vi "Measurement Logic.vi"() -> ()   [LabVIEW 2021, in "Efficiency_Class D Amplifier.lvlib"]
uses:
  Efficiency_Class D Amplifier.lvlib
  Measurement Configuration.ctl
  shared/controls/digital audio protocol/data justification.ctl
  shared/controls/digital audio protocol/endianness.ctl
  shared/controls/digital audio protocol/digital edge.ctl
  shared/controls/digital audio protocol/logic level.ctl
  shared/controls/digital output level units.ctl
  shared/controls/weighting filter.ctl
  shared/controls/lowpass filter.ctl
  shared/controls/highpass filter.ctl
  shared/controls/units - snr.ctl
  shared/controls/units - ratio.ctl
  shared/controls/power measurement method.ctl
  Measurement Results.ctl
  <vilib>/MeasurementLink/MeasurementLink Measurement Server/Measure Call Context/Measure Call Context.lvclass
  shared/controls/single tone measurement settings (HW).ctl
  <instrlib>/niDCPower/nidcpower.llb/niDCPower Source Mode.ctl
  <instrlib>/niDCPower/nidcpower.llb/niDCPower Output Function.ctl
  <instrlib>/niDMM/nidmm.llb/niDMM Function.ctl
  <instrlib>/niDMM/nidmm.llb/niDMM Resolution in Digits.ctl
  <instrlib>/niDMM/nidmm.llb/niDMM Configure Measurement Digits.vi
  <vilib>/PDM Acquisition Toolkit/host/Classes/Tasks/PCM Output/PCM Output Task.lvclass
  shared/controls/audio controls.lvlib
panel:
  out "Waveform Graph 2":cluster{"x0":dbl, "dx":dbl, "magnitude":dbl[]}(graph)
  out "Waveform Graph":waveform(dbl)(graph)
  in  "measurement configuration 2":T1={"digital channel list"="7821\\PCMo 8", "frame clock rate"=48000.0, "number of channels"=2, "channel length"=32, "bit depth"=24, "data justification"=enum."Left Justified", "endianness"=enum."MSB First", "bit clock edge sync"=enum."Rising", "frame sync edge for channel 0"=enum."Rising", "channel 0 offset"=1, "master clock channel list"="7821\\PCMo 0", "master clock rate"=12288000.0, "enable dither"=FALSE, "logic level"=enum."3.3 V", "signal frequency"=1000.0, "output level"=10.0, "output level units"=enum."% FS", "output range (pk-pk)"=15.0, "load impedance"=4.0, "signal phase"=0.0, "acq sampling rate"=51200.0, "min measurement cycles"=20, "min measurement time (s)"=0.1, "min settling cycles"=0, "min settling time (s)"=0.005, "acq channel"="PXI1Slot4/ai0", "band start"=20.0, "band stop"=20000.0, "weighting filter"=enum."Linear", "highpass filter"=enum."AC", "lowpass filter"=enum."No filter", "SNR units"=enum."dB", "THD+N units"=enum."dB", "THD units"=enum."dB", "gain units"=enum."dB"} {"acq sampling rate" format="%0.2f"; "master clock rate" format="%#_6pHz"; "frame clock rate" format="%#_6pHz"}
  out "measure call context out":refnum<class "Measure Call Context.lvclass">
  in  "measure call context in":refnum<class "Measure Call Context.lvclass">
  out "measurement results":T12={"channel name"="", "frequency (Hz)"=0.0, "amplitude (Vrms)"=0.0, "amplitude (dBFS)"=0.0, "THD+N"=0.0, "THD"=0.0, "power supply voltage (V)"=0.0, "power supply current (A)"=0.0, "input power (W)"=0.0, "output power (W)"=0.0, "power loss (W)"=0.0, "efficiency (%)"=0.0, "wfm - t0"=0.0, "wfm - dt"=1.9531249997269942e-05, "wfm - data"=array[12800 elements], "fft - f0"=0.0, "fft - df"=4.000000000559116, "fft - data"=array[6400 elements]}
  in  "measurement configuration":T13={"digital channel list"="7821\\PCMo 8", "frame clock rate"=48000.0, "number of channels"=2, "channel length"=32, "bit depth"=24, "data justification"=enum."Left Justified", "endianness"=enum."MSB First", "bit clock edge sync"=enum."Rising", "frame sync edge for channel 0"=enum."Rising", "channel 0 offset"=1, "master clock channel list"="7821\\PCMo 0", "master clock rate"=12288000.0, "enable dither"=FALSE, "logic level"=enum."3.3 V", "signal frequency"=1000.0, "output level"=1.0, "output level units"=enum."% FS", "output range (pk-pk)"=15.0, "load impedance"=4.0, "signal phase"=0.0, "acq sampling rate"=51200.0, "min measurement cycles"=20, "min measurement time (s)"=0.1, "min settling cycles"=0, "min settling time (s)"=0.005, "acq channel"="PXI1Slot4/ai0", "band start"=20.0, "band stop"=20000.0, "weighting filter"=enum."Linear", "lowpass filter"=enum."No filter", "highpass filter"=enum."DC", "SNR units"=enum."dB", "THD+N units"=enum."dB", "THD units"=enum."dB", "gain units"=enum."dB", "power measurement method"=enum."SMU", "power measurement resource"="PXI1Slot6/0", "power supply voltage"=14.4, "power supply current limit"=1.2, "sense resistor (Ohms)"=0.01} {"min settling cycles" format="%.3f"; "channel 0 offset" format="%#_6p"; "load impedance" format="%0.2f"; "acq sampling rate" format="%0.2f"; "frame clock rate" format="%#_6pHz"}
  out "error out":errorcluster
  in  "error in":errorcluster
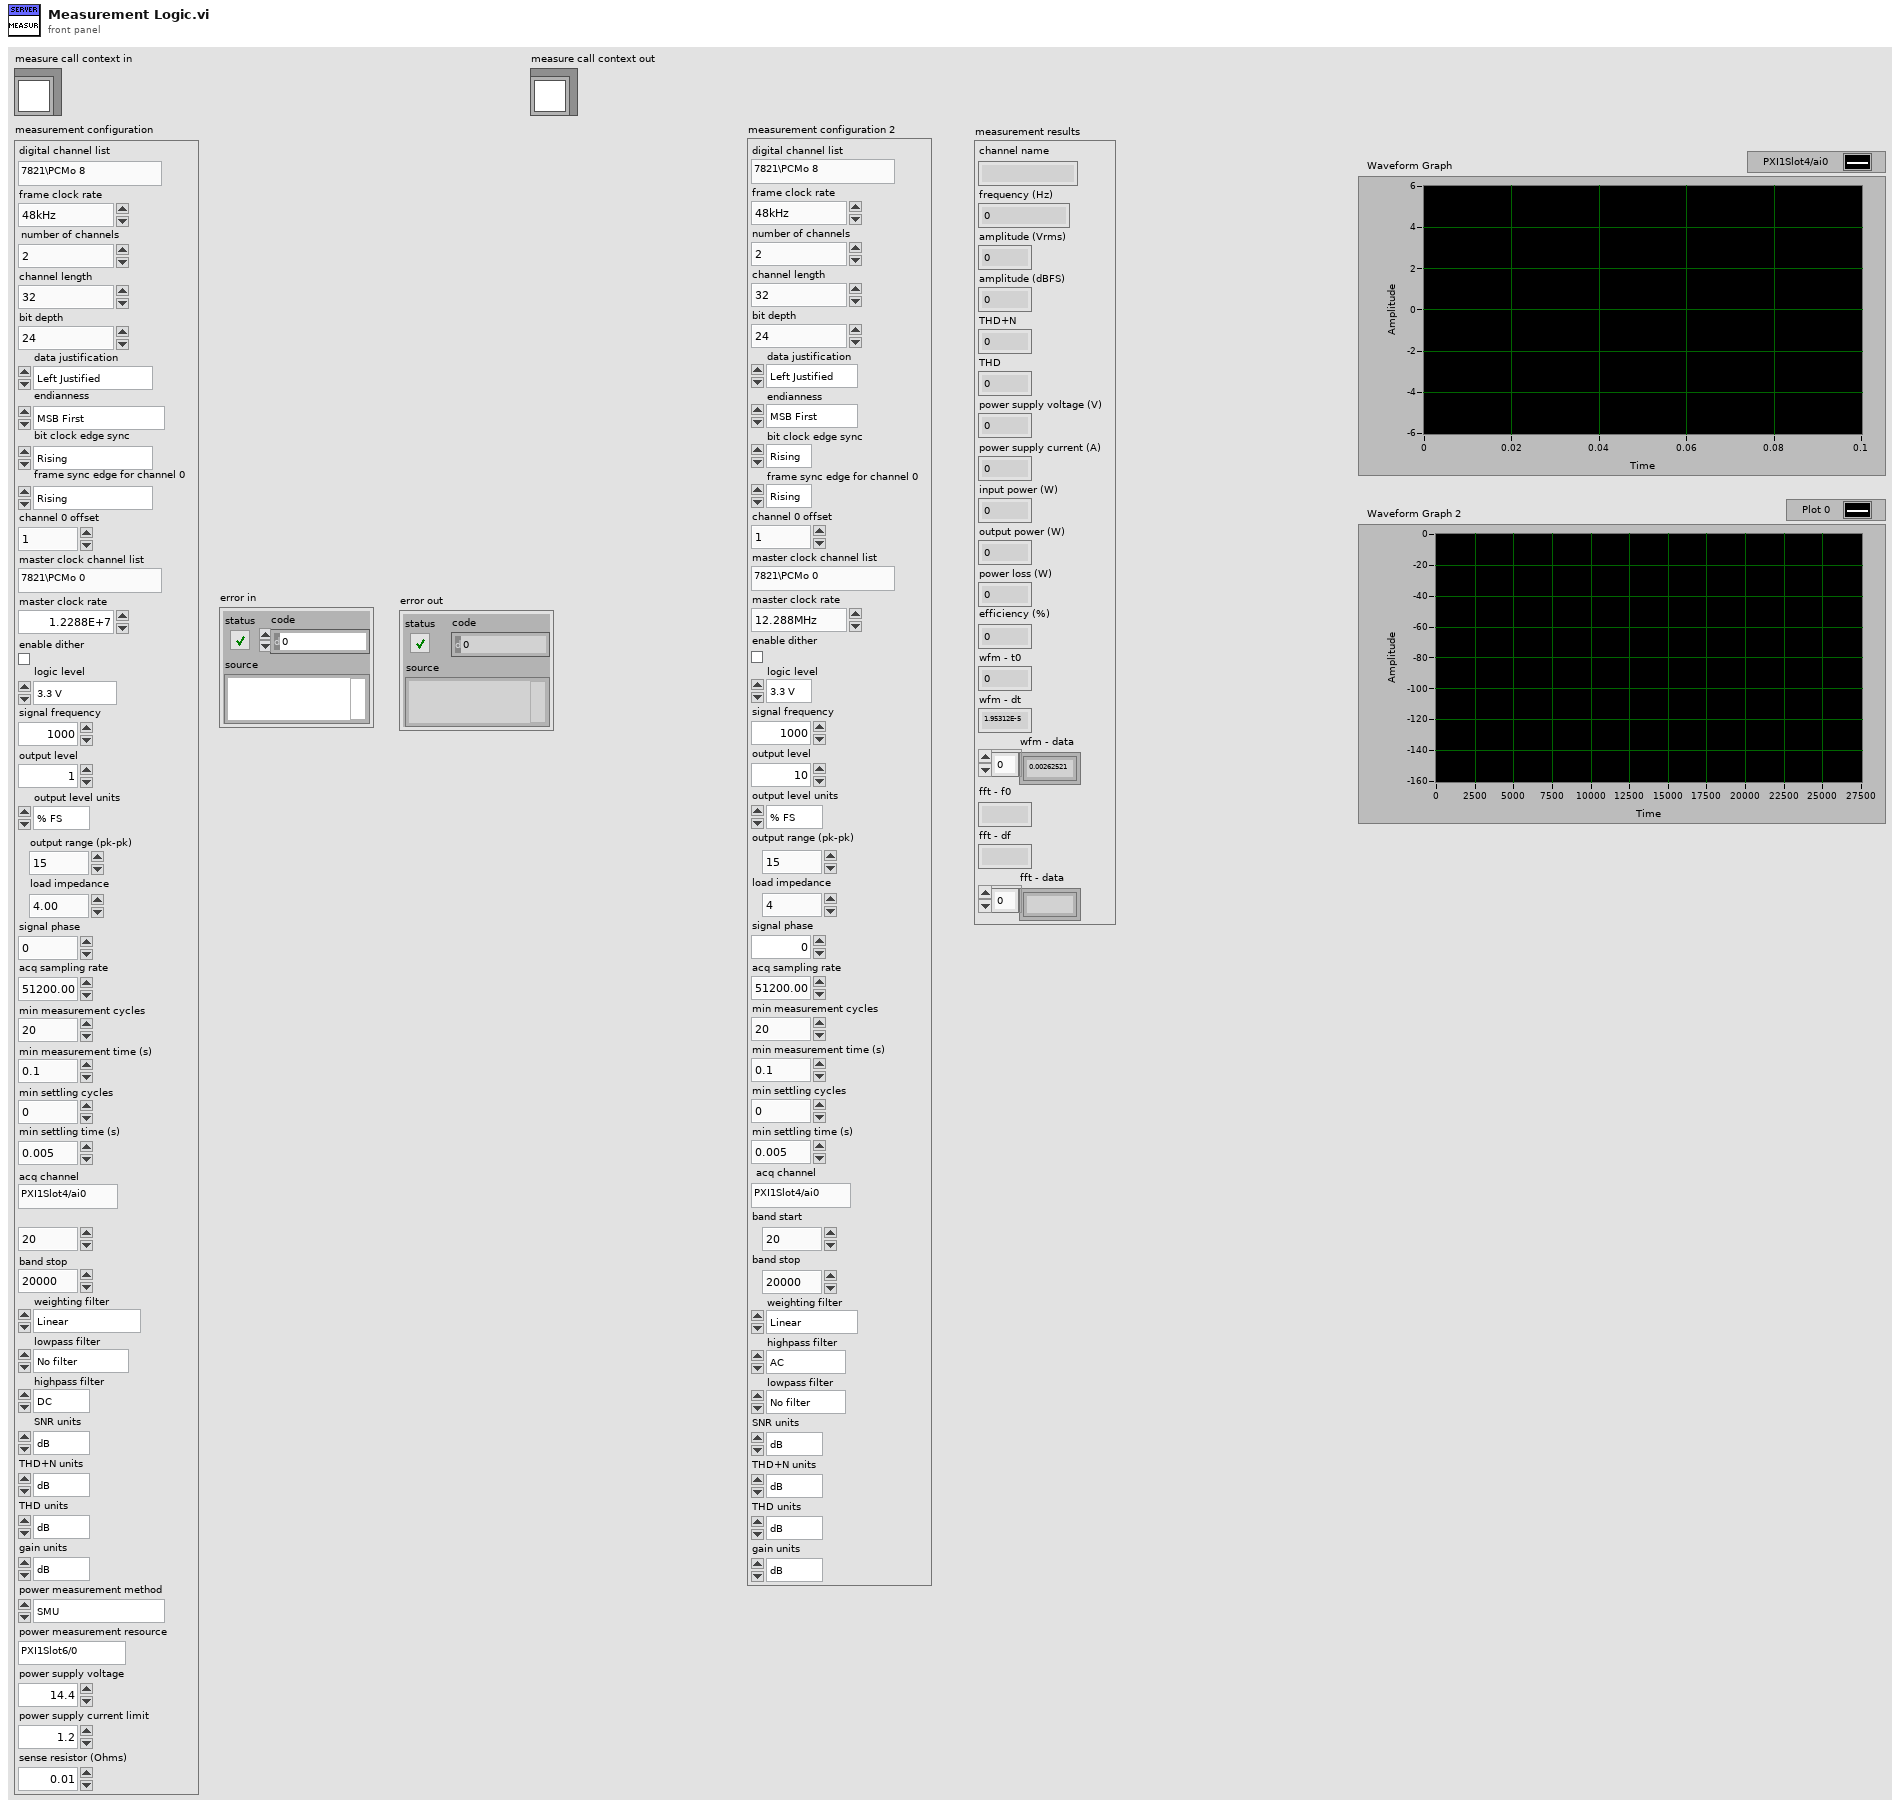
[diagram p1: front panel]
types:
  T1 = typedef "single tone measurement settings (HW).ctl" = cluster{"digital channel list":string, "frame clock rate":dbl, "number of channels":u32, "channel length":u32, "bit depth":u32, "data justification":T2, "endianness":T3, "bit clock edge sync":T4, "frame sync edge for channel 0":T4, "channel 0 offset":u32, "master clock channel list":string, "master clock rate":dbl, "enable dither":bool, "logic level":T5, "signal frequency":dbl, "output level":dbl, "output level units":T6, "output range (pk-pk)":dbl, "load impedance":dbl, "signal phase":dbl, "acq sampling rate":dbl, "min measurement cycles":u32, "min measurement time (s)":dbl, "min settling cycles":u32, "min settling time (s)":dbl, "acq channel":string, "band start":dbl, "band stop":dbl, "weighting filter":T7, "highpass filter":T8, "lowpass filter":T9, "SNR units":T10, "THD+N units":T11, "THD units":T11, "gain units":T11}
  T2 = typedef "data justification.ctl" = enum32{"Left Justified", "Right Justified"}
  T3 = typedef "endianness.ctl" = enum32{"MSB First", "LSB First"}
  T4 = typedef "digital edge.ctl" = enum32{"Rising", "Falling"}
  T5 = typedef "logic level.ctl" = enum32{"3.3 V", "1.8 V", "1.2 V"}
  T6 = typedef "audio controls.lvlib/digital output level units.ctl" = enum32{"% FS", "dBFS"}
  T7 = typedef "weighting filter.ctl" = enum32{"Linear", "A-weighting", "B-weighting", "C-weighting"}
  T8 = typedef "highpass filter.ctl" = enum32{"DC", "AC"}
  T9 = typedef "lowpass filter.ctl" = enum32{"No filter", "AES17 20kHz", "AES17 40kHz"}
  T10 = typedef "audio controls.lvlib/units - snr.ctl" = enum32{"dB", "x/y"}
  T11 = typedef "audio controls.lvlib/units - ratio.ctl" = enum32{"dB", "%", "x/y"}
  T12 = typedef "Efficiency_Class D Amplifier.lvlib/Measurement Results.ctl" = cluster{"channel name":string, "frequency (Hz)":dbl, "amplitude (Vrms)":dbl, "amplitude (dBFS)":dbl, "THD+N":dbl, "THD":dbl, "power supply voltage (V)":dbl, "power supply current (A)":dbl, "input power (W)":dbl, "output power (W)":dbl, "power loss (W)":dbl, "efficiency (%)":dbl, "wfm - t0":dbl, "wfm - dt":dbl, "wfm - data":dbl[], "fft - f0":dbl, "fft - df":dbl, "fft - data":dbl[]}
  T13 = typedef "Efficiency_Class D Amplifier.lvlib/Measurement Configuration.ctl" = cluster{"digital channel list":string, "frame clock rate":dbl, "number of channels":u32, "channel length":u32, "bit depth":u32, "data justification":T2, "endianness":T3, "bit clock edge sync":T4, "frame sync edge for channel 0":T4, "channel 0 offset":u32, "master clock channel list":string, "master clock rate":dbl, "enable dither":bool, "logic level":T5, "signal frequency":dbl, "output level":dbl, "output level units":T6, "output range (pk-pk)":dbl, "load impedance":dbl, "signal phase":dbl, "acq sampling rate":dbl, "min measurement cycles":u32, "min measurement time (s)":dbl, "min settling cycles":u32, "min settling time (s)":dbl, "acq channel":string, "band start":dbl, "band stop":dbl, "weighting filter":T7, "lowpass filter":T9, "highpass filter":T8, "SNR units":T10, "THD+N units":T11, "THD units":T11, "gain units":T11, "power measurement method":T14, "power measurement resource":string, "power supply voltage":dbl, "power supply current limit":dbl, "sense resistor (Ohms)":dbl}
  T14 = typedef "power measurement method.ctl" = enum16{"SMU", "DMM"}
  T15 = typedef "niDMM Function.ctl" = enum16{"DC Volts", "AC Volts", "DC Current", "AC Current", "2-wire Resistance", "4-wire Resistance", "Diode", "Frequency", "Period", "AC Volts DC Coupled", "Capacitance", "Inductance", "Temperature"}
  T16 = typedef "niDCPower Output Function.ctl" = i32
  T17 = typedef "niDCPower Source Mode.ctl" = i32
  T18 = typedef "niDMM Resolution in Digits.ctl" = dbl
  T19 = typedef "audio controls.lvlib/single tone audio measurements.ctl" = cluster{"channel":string, "frequency (Hz)":dbl, "amplitude (Vrms)":dbl, "amplitude (dBFS)":dbl, "phase (deg)":dbl, "SNR":dbl, "THD+N":dbl, "THD":dbl, "dynamic range (dB)":dbl, "gain":dbl, "SFDR (dBc)":dbl}
  T20 = typedef "PCM tasks.ctl" = cluster{"PCM output task":T21, "PCM output task-clock":T21}
  T21 = typedef "PDM Acquisition Class Library.lvlib/PCM Output Task.lvclass/PCM Output Task DVR.ctl" = refnum<data-value>
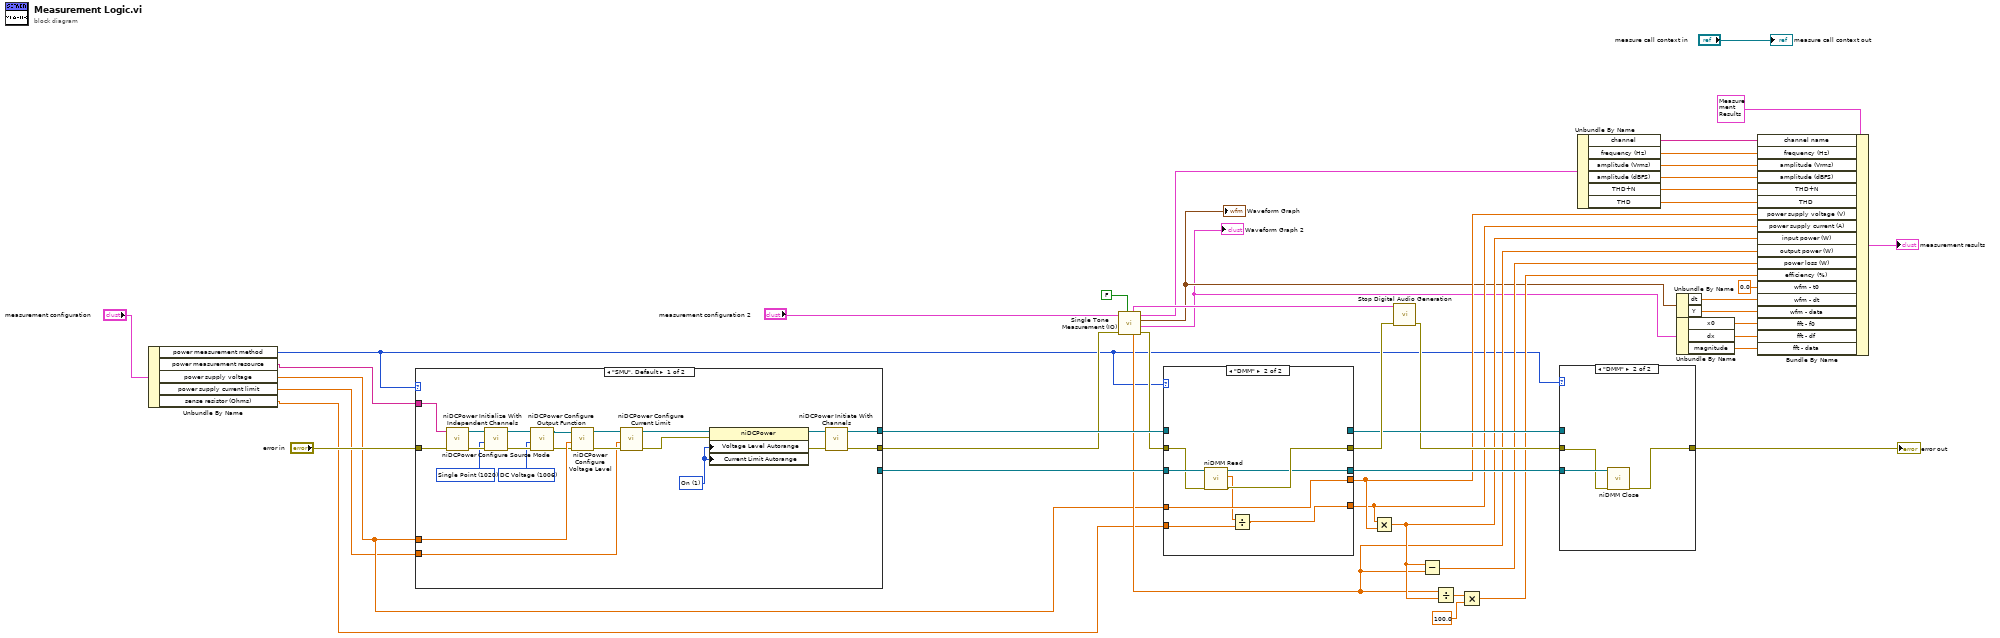
[diagram p0: block diagram]
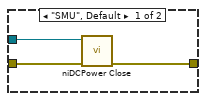
[diagram p2: hidden frame]
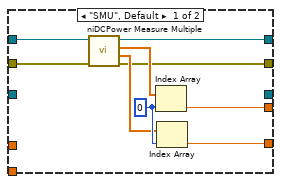
[diagram p3: hidden frame]
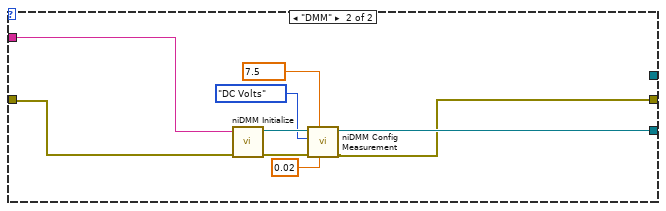
[diagram p4: hidden frame]
diagram:
  n1 = Unbundle By Name("measurement configuration") -> ("power measurement method"=w5:T14, "power measurement resource"=w4:string, "power supply voltage"=w3:dbl, "power supply current limit"=w2:dbl, "sense resistor (Ohms)"=w1:dbl)
  n2 = case shown="\"SMU\", Default" w5 {
    tunnel: w3 -> [w64 _]
    tunnel: w2 -> [w63 _]
    tunnel: [w49 _] -> w44
    tunnel: [w48 w71] -> w42
    tunnel: "error in" -> [w47 w75]
    tunnel: [_ w72] -> w33
    tunnel: w4 -> [w46 w67]
    frame "SMU", Default {
      w50 = 1 items=["Off", "On"] ("Source:DC Voltage:Current Limit Autorange")
      w51 = T16 1006 items=["DC Voltage"=1006, "DC Current"=1007, "Pulse Voltage"=1049, "Pulse Current"=1050] ("output function")
      w58 = T17 1020 items=["Single Point"=1020, "Sequence"=1021] ("source mode")
      n3 = call <instrlib>:"niDCPower Initialize With Independent Channels.vi"("error in (no error)"=w47, "resource name"=w46) -> ("error out"=w62:errorcluster, "instrument handle out"=w61:refnum<k15>)  [unwired: 8 in]
      n4 = call <instrlib>:"niDCPower Configure Source Mode.vi"("error in (no error)"=w62, "source mode"=w58, "instrument handle"=w61) -> ("error out"=w60:errorcluster, "instrument handle out"=w59:refnum<k15>)  [unwired: 7 out]
      n5 = call <instrlib>:"niDCPower Configure Output Function.vi"("error in (no error)"=w60, "output function"=w51, "instrument handle"=w59) -> ("error out"=w52:errorcluster, "instrument handle out"=w53:refnum<k15>)  [unwired: 1 in, 6 out]
      n6 = call <instrlib>:"niDCPower Configure Voltage Level.vi"("error in (no error)"=w52, "voltage level"=w64, "instrument handle"=w53) -> ("error out"=w65:errorcluster, "instrument handle out"=w66:refnum<k15>)  [unwired: 1 in, 6 out]
      n7 = call <instrlib>:"niDCPower Configure Current Limit.vi"("error in (no error)"=w65, "current limit"=w63, "instrument handle"=w66) -> ("error out"=w54:errorcluster, "instrument handle out"=w57:refnum<k15>)  [unwired: 2 in, 5 out]
      n8 = property class="niDCPower"(reference=w57, error in=w54, "Voltage Level Autorange"=w50, "Current Limit Autorange"=w50) -> (reference out=w56:refnum<k15>, error out=w55:errorcluster)
      n9 = call <instrlib>:"niDCPower Initiate With Channels.vi"("error in (no error)"=w55, "instrument handle"=w56) -> ("error out"=w48:errorcluster, "instrument handle out"=w49:refnum<k15>)  [unwired: 8 in]
    }
    frame "DMM" {
      w69 = T18 7.5 items=["3 1/2"=3.5, "4 1/2"=4.5, "5 1/2"=5.5, "6 1/2"=6.5, "7 1/2"=7.5] ("Resolution in Digits")
      n10 = call <instrlib>:"niDMM Initialize.vi"("error in (no error)"=w75, "Instrument Descriptor"=w67) -> ("error out"=w74:errorcluster, "instrument handle out"=w73:refnum<k15>)  [unwired: 8 in]
      n11 = call-poly <instrlib>:"niDMM Config Measurement.vi"("Range"=0.02, "Resolution in Digits"=w69, "error in (no error)"=w74, "Function"=niDMM_Function."DC Volts", "instrument handle"=w73) -> ("error out"=w71:errorcluster, "instrument handle out"=w72:refnum<k15>)  [unwired: 5 in]
    }
  }
  n12 = call "Single Tone Measurement (IO).vi"("stop generation"=FALSE, "error in (no error)"=w42, "measurement configuration"="measurement configuration 2") -> ("error out"=w37:errorcluster, "spectrum"=w10:cluster{"x0":dbl, "dx":dbl, "magnitude":dbl[]}, "time domain"=w11:waveform(dbl), "results"=w27:T19, "output power"=w17:dbl, "PCM tasks"=w35:T20)  [unwired: 3 in]
  "Waveform Graph" <- w11
  "Waveform Graph 2" <- w10
  n13 = case shown="\"DMM\"" w5 {
    tunnel: w44 -> [w84 _]
    tunnel: [w83 _] -> w32
    tunnel: [w82 w89] -> w20
    tunnel: [w81 w86] -> w19
    tunnel: [w77 w90] -> w38
    tunnel: w37 -> [w76 w91]
    tunnel: w33 -> [_ w92]
    tunnel: w1 -> [_ w87]
    tunnel: w3 -> [_ w89]
    tunnel: [_ w85] -> w30
    frame "SMU", Default {
      w80 = 0 ("index")
      n14 = call <instrlib>:"niDCPower Measure Multiple.vi"("error in (no error)"=w76, "instrument handle"=w84) -> ("error out"=w77:errorcluster, "current measurements"=w78:dbl[], "voltage measurements"=w79:dbl[], "instrument handle out"=w83:refnum<k15>)  [unwired: 6 in]
      n15 = Index Array(array=w79, index=w80) -> (element=w82:dbl)
      n16 = Index Array(array=w78, index=w80) -> (element=w81:dbl)
    }
    frame "DMM" {
      n17 = call <instrlib>:"niDMM Read.vi"("error in (no error)"=w91, "instrument handle"=w92) -> ("error out"=w90:errorcluster, "Measurement"=w88:dbl, "instrument handle out"=w85:refnum<k15>)  [unwired: 7 in]
      n18 = Divide(x=w88, y=w87) -> (x/y=w86:dbl)
    }
  }
  n19 = Multiply(x=w19, y=w20) -> (x*y=w18:dbl)
  n20 = call "Stop Digital Audio Generation.vi"("error in (no error)"=w38, "PCM tasks"=w35) -> ("error out"=w31:errorcluster)  [unwired: 9 in]
  n21 = Subtract(x=w18, y=w17) -> (x-y=w16:dbl)
  n22 = Divide(x=w17, y=w18) -> (x/y=w40:dbl)
  n23 = Multiply(x=w40, y=100.0) -> (x*y=w15:dbl)
  n24 = case shown="\"DMM\"" w5 {
    tunnel: [w95 w96] -> w43
    tunnel: w32 -> [w94 _]
    tunnel: w31 -> [w93 w97]
    tunnel: w30 -> [_ w98]
    frame "SMU", Default {
      n25 = call <instrlib>:"niDCPower Close.vi"("error in (no error)"=w93, "instrument handle"=w94) -> ("error out"=w95:errorcluster)  [unwired: 9 out]
    }
    frame "DMM" {
      n26 = call <instrlib>:"niDMM Close.vi"("error in (no error)"=w97, "instrument handle"=w98) -> ("error out"=w96:errorcluster)  [unwired: 9 in]
    }
  }
  "error out" <- w43
  n27 = Unbundle By Name(w27) -> ("channel"=w26:string, "frequency (Hz)"=w25:dbl, "amplitude (Vrms)"=w24:dbl, "amplitude (dBFS)"=w23:dbl, "THD+N"=w22:dbl, "THD"=w21:dbl)
  n28 = Unbundle By Name(w11) -> ("dt"=w14:dbl, "Y"=w13:dbl[])
  n29 = Unbundle By Name(w10) -> ("x0"=w9:dbl, "dx"=w8:dbl, "magnitude"=w7:dbl[])
  n30 = Bundle By Name(cluster=T12 {"channel name"="", "frequency (Hz)"=0.0, "amplitude (Vrms)"=0.0, "amplitude (dBFS)"=0.0, "THD+N"=0.0, "THD"=0.0, "power supply voltage (V)"=0.0, "power supply current (A)"=0.0, "input power (W)"=0.0, "output power (W)"=0.0, "power loss (W)"=0.0, "efficiency (%)"=0.0, "wfm - t0"=0.0, "wfm - dt"=1.9531249997269942e-05, "wfm - data"=array[12800 elements], "fft - f0"=0.0, "fft - df"=4.000000000559116, "fft - data"=array[6400 elements]} ("measurement results"), "channel name"=w26, "frequency (Hz)"=w25, "amplitude (Vrms)"=w24, "amplitude (dBFS)"=w23, "THD+N"=w22, "THD"=w21, "power supply voltage (V)"=w20, "power supply current (A)"=w19, "input power (W)"=w18, "output power (W)"=w17, "power loss (W)"=w16, "efficiency (%)"=w15, "wfm - t0"=0.0, "wfm - dt"=w14, "wfm - data"=w13, "fft - f0"=w9, "fft - df"=w8, "fft - data"=w7) -> (→"measurement results":T12)
  "measure call context out" <- "measure call context in"
